vi "Get Compiled Counter And Protection Frames.vi"(0 "XNET Cluster":refnum<k21>, 5 "GUIDs":T9, 7 "Frames per type":T10[](array[typedef]) {"Frame Settings"."Tx Control.Override Period Value Ref" format="%.0x"; "Frame Settings"."Tx Control.Override Period Ref" format="%.0x"; "Frame Settings"."Tx Control.Disable Tx Ref" format="%.0x"; "Frame Settings"."Transmit Trigger Ref" format="%.0x"; "Frame Settings"."Disable Transmission Ref" format="%.0x"; "Frame Refs" format="%.0x"}, 11 "error in (no error)":errorcluster) -> (4 "Frames":T2[](array[typedef]) {"Protection Configurations"."CRC Channels"."Data Type" items=["Signed", "Unsigned", "IEEE Float"]}, 6 "Signals Refs":T1[](array[typedef]) format="%.0x", 8 "Counters and Protection Refs":T1[](array[typedef]) format="%.0x", 10 "Override Refs":T1[](array[typedef]) format="%.0x", 15 "error out":errorcluster)   [LabVIEW 2023, in "Protection and Counter Support System Explorer.lvlib"]
uses:
  Protection and Counter Support System Explorer.lvlib
  Types/Export Frames List and Type.ctl
  Shared/Types/Exported Frame Type.ctl
  <vilib>/NI VeriStand/Custom Device API/Custom Device Item Ref.ctl
  Types/Exported Frame Settings.ctl
  Shared/Types/Exported Event Trigger Type.ctl
  Types/Export Frame GUIDs List.ctl
  Shared/Types/Exported Frame Settings.ctl
  Shared/Types/Exported Protection Settings.ctl
  Shared/Types/Protection Type.ctl
  Shared/Types/XNET Signal Configuration.ctl
  Shared/Types/Exported Counter Settings.ctl
  <vilib>/NI VeriStand/Custom Device Tools/Custom Device Utility Library/NI VeriStand - Search for All Items by GUID.vi
  Shared/Protection and Counter Support Shared.lvlib
  <vilib>/NI VeriStand/Custom Device API/Custom Device API.lvlib
  <resource>/objmgr/xnet.rc
  <vilib>/NI VeriStand/Custom Device Tools/Custom Device Utility Library/Custom Device Utility Library.lvlib
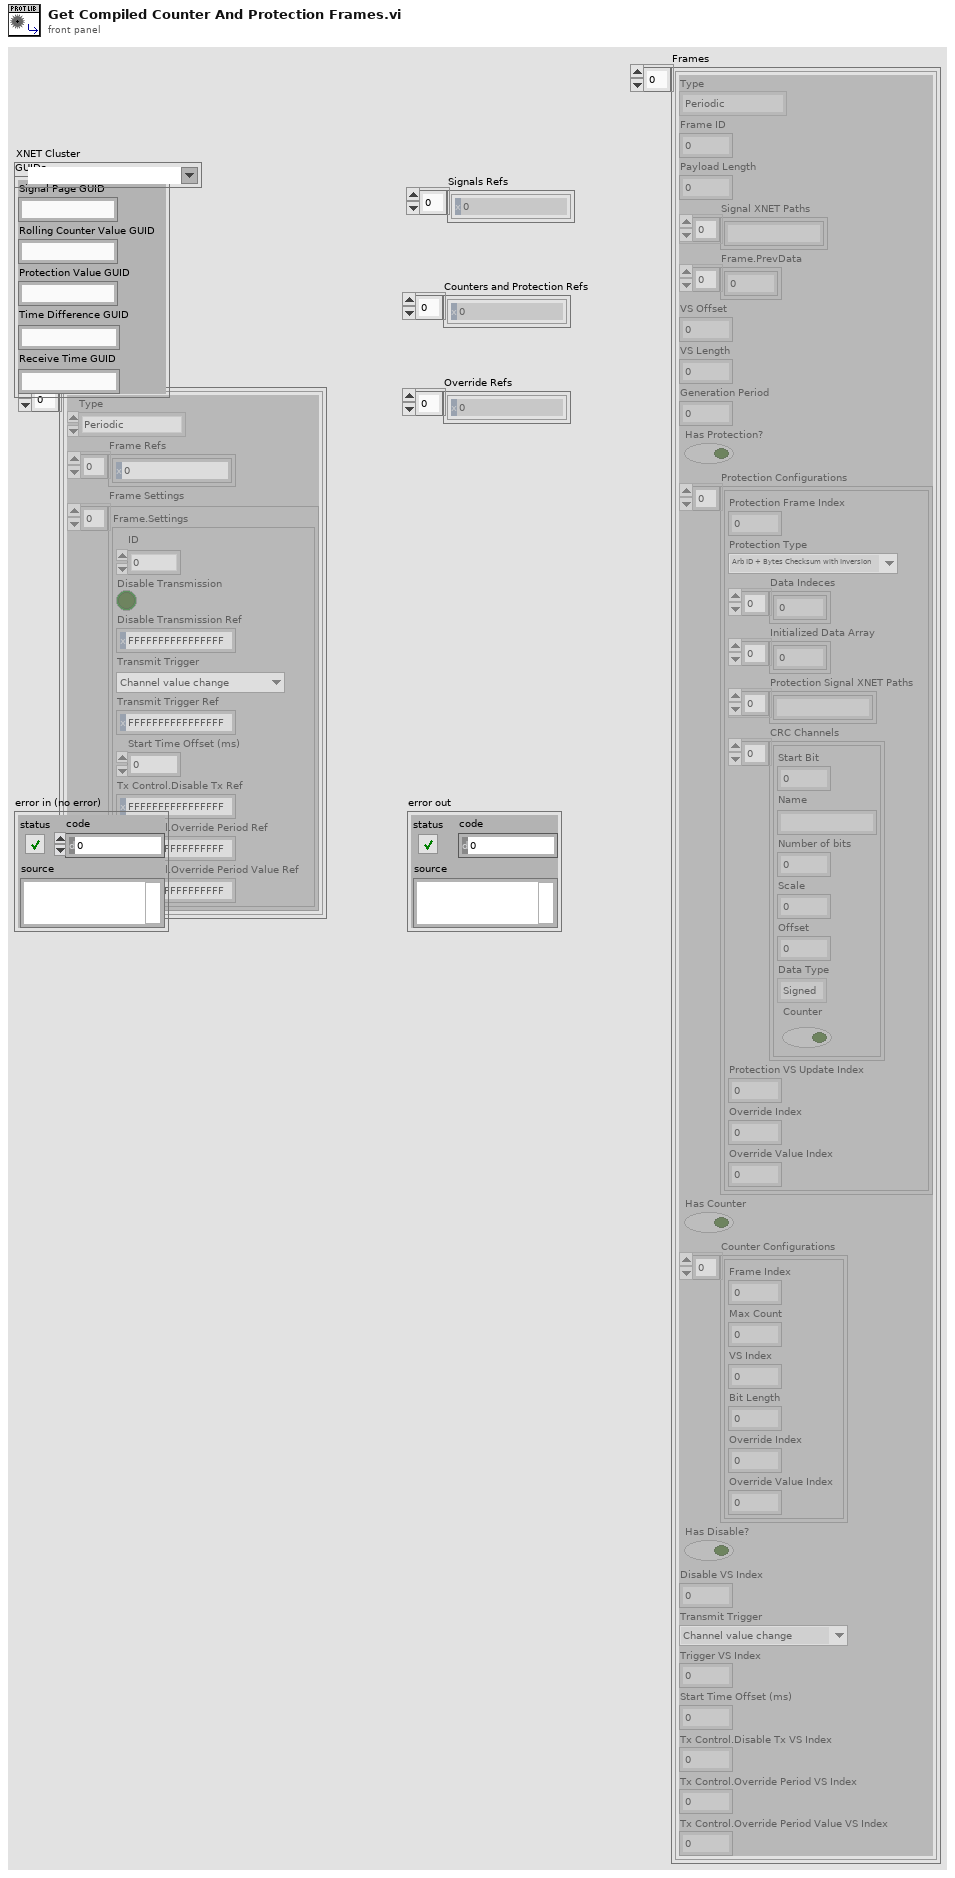
[diagram p1: front panel]
types:
  T1 = typedef "Custom Device API.lvlib/Custom Device Item Ref.ctl" = u64
  T2 = typedef "Protection and Counter Support Shared.lvlib/Exported Frame Settings.ctl" = cluster{"Type":T3, "Frame ID":u32, "Payload Length":u32, "Signal XNET Paths":string[], "Frame.PrevData":dbl[], "VS Offset":i32, "VS Length":i32, "Generation Period":u32, "Has Protection?":bool, "Protection Configurations":T4[], "Has Counter":bool, "Counter Configurations":T7[], "Has Disable?":bool, "Disable VS Index":i32, "Transmit Trigger":T8, "Trigger VS Index":i32, "Start Time Offset (ms)":u32, "Tx Control.Disable Tx VS Index":i32, "Tx Control.Override Period VS Index":i32, "Tx Control.Override Period Value VS Index":i32}
  T3 = typedef "Protection and Counter Support Shared.lvlib/Exported Frame Type.ctl" = enum16{"Periodic", "Event", "Periodic/Event"}
  T4 = typedef "Protection and Counter Support Shared.lvlib/Exported Protection Settings.ctl" = cluster{"Protection Frame Index":i32, "Protection Type":T5, "Data Indeces":i32[], "Initialized Data Array":dbl[], "Protection Signal XNET Paths":string[], "CRC Channels":T6[], "Protection VS Update Index":i32, "Override Index":i32, "Override Value Index":i32}
  T5 = typedef "Protection and Counter Support Shared.lvlib/Protection Type.ctl" = enum16{"Arb ID + Bytes Checksum with Inversion", "Arb ID + Bytes CRC with Inversion", "Reversed Raw Signal Checksum with Inversion", "Concatenated Two's Compliment", "LP_CRC8", "LP_Checksum", "LP_CRC8_MRS"}
  T6 = typedef "Protection and Counter Support Shared.lvlib/XNET Signal Configuration.ctl" = cluster{"Start Bit":i32, "Name":string, "Number of bits":i32, "Scale":dbl, "Offset":dbl, "Data Type":u32, "Counter":bool}
  T7 = typedef "Protection and Counter Support Shared.lvlib/Exported Counter Settings.ctl" = cluster{"Frame Index":i32, "Max Count":dbl, "VS Index":i32, "Bit Length":i64, "Override Index":i32, "Override Value Index":i32}
  T8 = typedef "Protection and Counter Support Shared.lvlib/Exported Event Trigger Type.ctl" = enum16{"Channel value change", "Trigger channel (not zero)", "Channel value change or trigger channel (not zero)", "Trigger channel (any value change)", "Channel value change or trigger channel (any value change)"}
  T9 = typedef "Protection and Counter Support System Explorer.lvlib/Export Frame GUIDs List.ctl" = cluster{"Signal Page GUID":string, "Rolling Counter Value GUID":string, "Protection Value GUID":string, "Time Difference GUID":string, "Receive Time GUID":string}
  T10 = typedef "Protection and Counter Support System Explorer.lvlib/Export Frames List and Type.ctl" = cluster{"Type":T3, "Frame Refs":T1[], "Frame Settings":T11[]}
  T11 = typedef "Protection and Counter Support System Explorer.lvlib/Exported Frame Settings.ctl" = cluster{"ID":u32, "Disable Transmission":bool, "Disable Transmission Ref":T1, "Transmit Trigger":T8, "Transmit Trigger Ref":T1, "Start Time Offset (ms)":u32, "Tx Control.Disable Tx Ref":T1, "Tx Control.Override Period Ref":T1, "Tx Control.Override Period Value Ref":T1}
  T12 = typedef "Custom Device API.lvlib/Custom Device Item Info.ctl" = cluster{"Name":string, "Is Channel":bool, "GUID":string, "Is Waveform":bool}
  T13 = typedef "Protection and Counter Support System Explorer.lvlib/Protection Signal Settings.ctl" = cluster{"Input Channels":T14[], "Protection Type":T5}
  T14 = typedef "Protection and Counter Support System Explorer.lvlib/Protection Signal Linked Channel.ctl" = cluster{"Node Ref":T1}
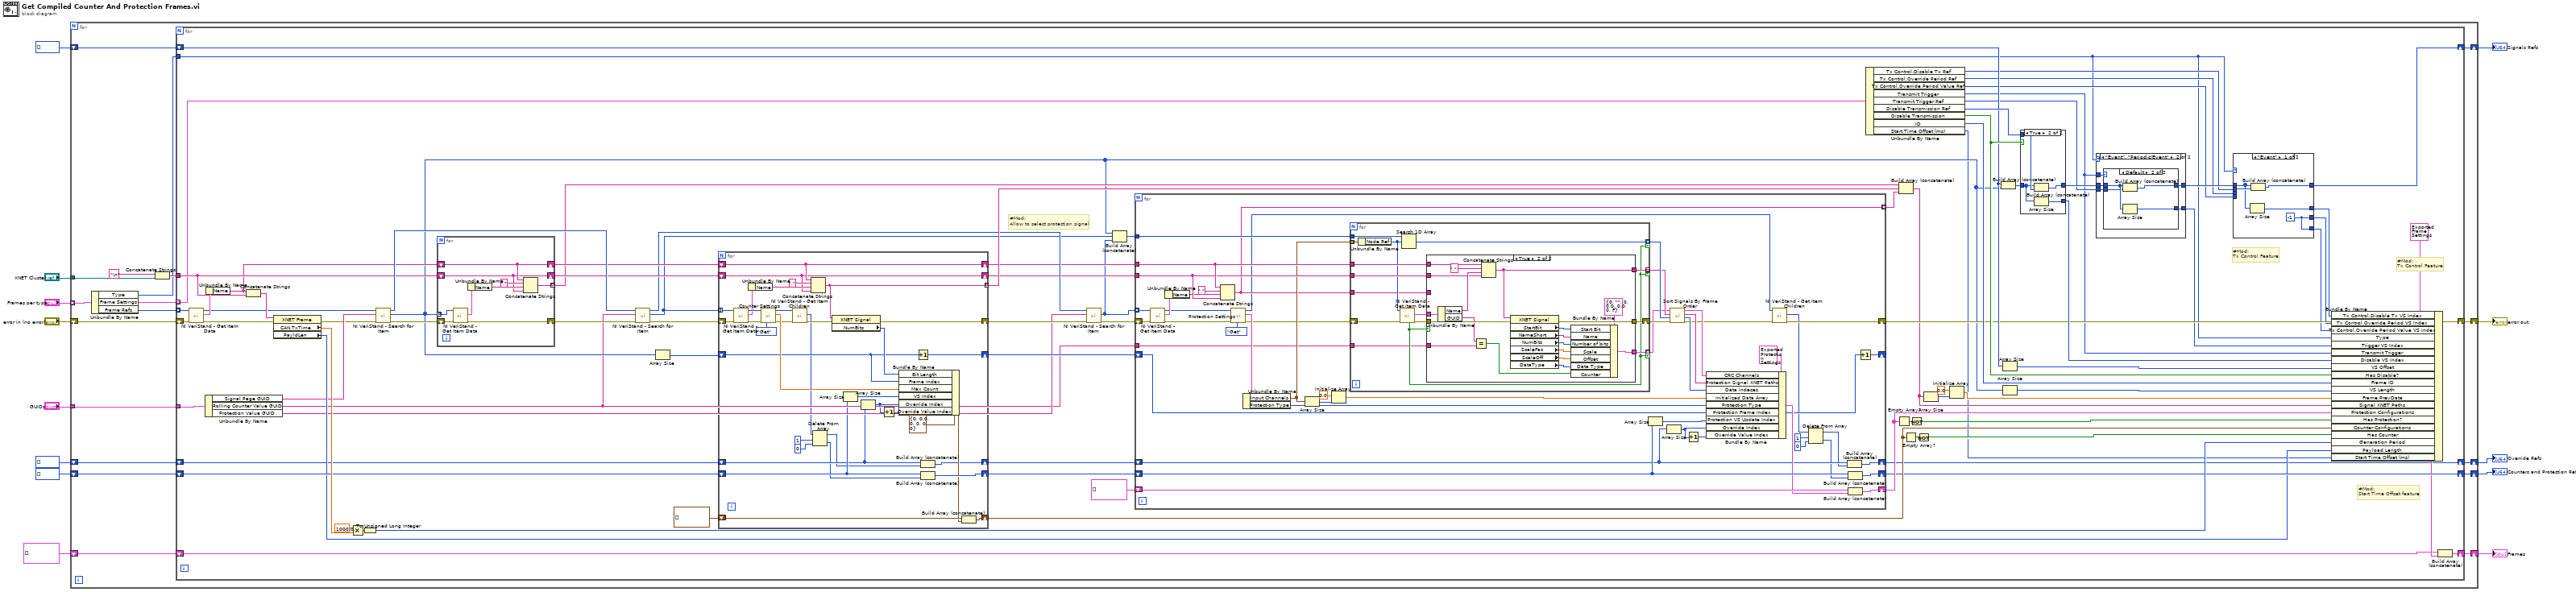
[diagram p0: block diagram]
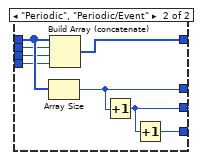
[diagram p2: hidden frame]
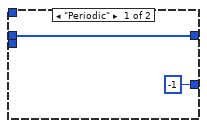
[diagram p3: hidden frame]
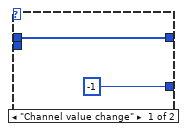
[diagram p4: hidden frame]
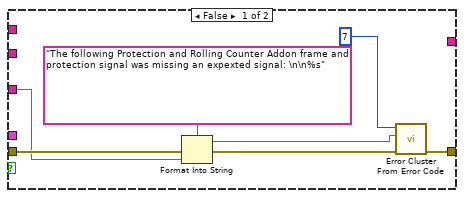
[diagram p5: hidden frame]
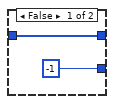
[diagram p6: hidden frame]
diagram:
  n1 = for {
    tunnel: "XNET Cluster" -> [w31]
    shift-right: [w26] -> w1
    shift-left: "error in (no error)" -> [w20]
    shift-right: [w25] -> w7
    shift-left: T2[] [] -> [w24]
    shift-right: [w28] -> w5
    shift-left: T1[] [] -> [w23]
    shift-right: [w27] -> w6
    shift-left: T1[] [] -> [w22]
    tunnel: "GUIDs" -> [w21]
    tunnel: "Frames per type" -> [w19] mode=indexing
    shift-right: [w14] -> w2
    shift-left: T1[] [] -> [w15]
    n2 = Unbundle By Name(w19) -> ("Type"=w18:T3, "Frame Settings"=w16:T11[], "Frame Refs"=w17:T1[])
    n3 = Concatenate Strings("\n", w31) -> (w29:string)
    n4 = for {
      tunnel: w17 -> [w99] mode=indexing
      shift-right: [w69] -> w26
      shift-left: w20 -> [w100]
      shift-right: [w37] -> w28
      shift-left: w23 -> [w109]
      tunnel: w29 -> [w84]
      shift-right: [w63] -> w27
      shift-left: w22 -> [w90]
      shift-right: [w54] -> w25
      shift-left: w24 -> [w53]
      tunnel: w18 -> [w36]
      tunnel: w21 -> [w52]
      tunnel: w16 -> [w49] mode=indexing
      shift-right: [w44] -> w14
      shift-left: w15 -> [w46]
      # "#Mod:\nTx Control Feature"
      # "#Mod:\nTx Control Feature"
      # "#Mod:\nAllow to select protection signal"
      # "#Mod:\nStart Time Offset feature"
      n5 = call <vilib>:"NI VeriStand - Get Item Data.vi"("error in (no error)"=w100, "Item Ref in"=w99) -> ("error out"=w96:errorcluster, "Item Info"=w98:T12, "Item Ref out"=w32:T1)  [unwired: 6 in, 1 out]
      n6 = Unbundle By Name(w52) -> ("Signal Page GUID"=w51:string, "Rolling Counter Value GUID"=w47:string, "Protection Value GUID"=w50:string)
      n7 = Unbundle By Name(w98) -> ("Name"=w83:string)
      n8 = Concatenate Strings(w83, w84) -> (w97:string)
      n9 = property class="XNET Frame"(reference=w97, error in=w96) -> (error out=w48:errorcluster, "CAN.TxTime"=w94:dbl, "PayldLen"=w59:u32)  [unwired: 1 out]
      n10 = Multiply(x=1000.0 ("y"), y=w94) -> (x*y=w95:dbl)
      n11 = To Unsigned Long Integer(number=w95) -> (unsigned 32bit integer=w92:u32)
      n12 = call-poly <vilib>:"NI VeriStand - Search for Item.vi"("error in"=w48, "Item GUID"=w51, "Section Ref in"=w32) -> ("error out"=w86:errorcluster, "Item Refs"=w61:T1[], "Section Ref out"=w89:T1)  [unwired: 5 in, 1 out]
      n13 = for {
        tunnel: w61 -> [w239] mode=indexing
        shift-right: [w233] -> w85
        shift-left: w86 -> [w238]
        tunnel: [w235] -> w80 mode=indexing
        shift-right: [w232] -> w82
        shift-left: w83 -> [w232]
        shift-right: [w231] -> w81
        shift-left: w84 -> [w231]
        n14 = call <vilib>:"NI VeriStand - Get Item Data.vi"("error in (no error)"=w238, "Item Ref in"=w239) -> ("error out"=w233:errorcluster, "Item Info"=w234:T12)  [unwired: 6 in, 2 out]
        n15 = Unbundle By Name(w234) -> ("Name"=w236:string)
        n16 = Concatenate Strings(w232, "." ("string"), w236, w231) -> (w235:string)
      }
      n17 = call-poly <vilib>:"NI VeriStand - Search for Item.vi"("error in"=w85, "Item GUID"=w47, "Section Ref in"=w89) -> ("error out"=w88:errorcluster, "Item Refs"=w60:T1[], "Section Ref out"=w77:T1)  [unwired: 5 in, 1 out]
      n18 = Array Size(array=w61) -> (size(s)=w87:i32)
      n19 = for {
        tunnel: w60 -> [w274] mode=indexing
        shift-right: [w255] -> w78
        shift-left: w88 -> [w273]
        shift-right: [w270] -> w101
        shift-left: T7[] [] -> [w269]
        tunnel: [w254] -> w79 mode=indexing
        shift-right: [w264] -> w64
        shift-left: w90 -> [w265]
        shift-right: [w259] -> w74
        shift-left: w87 -> [w252]
        shift-right: [w258] -> w72
        shift-left: w82 -> [w258]
        shift-right: [w257] -> w73
        shift-left: w81 -> [w257]
        shift-right: [w246] -> w45
        shift-left: w46 -> [w251]
        n20 = call <vilib>:"NI VeriStand - Get Item Data.vi"("error in (no error)"=w273, "Item Ref in"=w274) -> ("error out"=w271:errorcluster, "Item Info"=w266:T12, "Item Ref out"=w272:T1)  [unwired: 6 in, 1 out]
        n21 = Unbundle By Name(w266) -> ("Name"=w267:string)
        n22 = call "Counter Settings.vi"("Action"=enum8{"Get", "Set"}."Get", "error in"=w271, "Parent Ref"=w272) -> ("error out"=w248:errorcluster, "Max Count"=w263:dbl, "Parent Ref Out"=w243:T1)  [unwired: 6 in]
        n23 = call <vilib>:"NI VeriStand - Get Item Children.vi"("error in (no error)"=w248, "Item Ref in"=w243) -> ("error out"=w247:errorcluster, "Child Refs"=w241:T1[])  [unwired: 6 in, 2 out]
        n24 = Concatenate Strings(w258, "." ("string"), w267, w257) -> (w254:string)
        n25 = Delete From Array(array=w241, length=1, index=0) -> (deleted portion=w242:T1[], array with subset deleted=w240:T1[])
        n26 = property class="XNET Signal"(reference=w254, error in=w247) -> (error out=w255:errorcluster, "NumBits"=w253:u32)  [unwired: 1 out]
        n27 = Array Size(array=w265) -> (size(s)=w260:i32)
        n28 = Array Size(array=w251) -> (size(s)=w250:i32)
        n29 = Increment(x=w250) -> (x+1=w249:i32)
        n30 = Bundle By Name(cluster=T7 {"Frame Index"=0, "Max Count"=0.0, "VS Index"=0, "Bit Length"=0, "Override Index"=0, "Override Value Index"=0} ("Cluster"), "Bit Length"=w253, "Frame Index"=w252, "Max Count"=w263, "VS Index"=w260, "Override Index"=w250, "Override Value Index"=w249) -> (w262:T7)
        n31 = Increment(x=w252) -> (x+1=w259:i32)
        n32 = Build Array (concatenate)(w251, w240) -> (w246:T1[])
        n33 = Build Array (concatenate)(w265, w242) -> (w264:T1[])
        n34 = Build Array (concatenate)(w269, w262) -> (w270:T7[])
      }
      n35 = call-poly <vilib>:"NI VeriStand - Search for Item.vi"("error in"=w78, "Item GUID"=w50, "Section Ref in"=w77) -> ("error out"=w76:errorcluster, "Item Refs"=w42:T1[])  [unwired: 5 in, 2 out]
      n36 = Build Array (concatenate)(w61, w60, w42) -> (w62:T1[])
      n37 = for {
        tunnel: w42 -> [w189] mode=indexing
        shift-right: [w148] -> w69
        shift-left: w76 -> [w188]
        shift-right: [w185] -> w70
        shift-left: T4[] [] -> [w187]
        tunnel: w62 -> [w186]
        tunnel: w72 -> [w183]
        tunnel: [w165] -> w71 mode=indexing
        shift-right: [w179] -> w63
        shift-left: w64 -> [w180]
        shift-right: [w167] -> _
        shift-left: w74 -> [w168]
        tunnel: w73 -> [w182]
        tunnel: w47 -> [w163]
        shift-right: [w153] -> w44
        shift-left: w45 -> [w152]
        n38 = call <vilib>:"NI VeriStand - Get Item Data.vi"("error in (no error)"=w188, "Item Ref in"=w189) -> ("error out"=w151:errorcluster, "Item Info"=w181:T12, "Item Ref out"=w150:T1)  [unwired: 6 in, 1 out]
        n39 = Unbundle By Name(w181) -> ("Name"=w166:string)
        n40 = Concatenate Strings(w183, "." ("string"), w166, w182) -> (w165:string)
        n41 = call "Protection Settings.vi"("Action"=enum8{"Get", "Set"}."Get", "error in"=w151, "Parent Ref"=w150) -> ("error out"=w171:errorcluster, "Selected Channels"=w178:T13, "Parent Ref Out"=w147:T1)  [unwired: 6 in]
        n42 = Unbundle By Name(w178) -> ("Input Channels"=w176:T14[], "Protection Type"=w177:T5)
        n43 = Array Size(array=w176) -> (size(s)=w175:i32)
        n44 = Initialize Array(0.0 ("element"), w175) -> (w173:dbl[])
        n45 = for {
          tunnel: w186 -> [w194]
          tunnel: w176 -> [w204] mode=indexing
          tunnel: [w203] -> w162 mode=indexing if=w192
          shift-right: [w197] -> w160
          shift-left: w171 -> [w202]
          tunnel: w183 -> [w200]
          tunnel: w182 -> [w199]
          tunnel: [w195] -> w159 mode=indexing if=w192
          tunnel: [w196] -> w158 mode=indexing if=w192
          tunnel: w165 -> [w191]
          tunnel: w163 -> [w190]
          n46 = Unbundle By Name(w204) -> ("Node Ref"=w193:T1)
          n47 = call <vilib>:"NI VeriStand - Get Item Data.vi"("error in (no error)"=w202, "Item Ref in"=w193) -> ("error out"=w198:errorcluster, "Item Info"=w201:T12, "Found"=w192:bool)  [unwired: 6 in, 1 out]
          n48 = Search 1D Array(1D array=w194, element=w193) -> (index of element=w203:i32)  [unwired: 1 in]
          n49 = case shown="True" w192 {
            tunnel: w201 -> [_ w230]
            tunnel: w200 -> [_ w227]
            tunnel: w199 -> [_ w226]
            tunnel: w198 -> [w209 w225]
            tunnel: [w211 w224] -> w197
            tunnel: [_ w216] -> w196
            tunnel: [_ w212] -> w195
            tunnel: w191 -> [w206 _]
            tunnel: w190 -> [_ w215]
            frame False {
              n50 = Format Into String(format string="The following Protection and Rolling Counter Addon frame and protection signal was missing an expexted signal: \n\n%s" ("error message (\"\")"), error in=w209, w206) -> (resulting string=w205:string, error out=w208:errorcluster)  [unwired: 1 in]
              n51 = call <vilib>:"Error Cluster From Error Code.vi"("error in (no error)"=w208, "error message (\"\")"=w205, "error code (0)"=7) -> ("error out"=w211:errorcluster)  [unwired: 6 in]
            }
            frame True {
              n52 = Unbundle By Name(w230) -> ("Name"=w228:string, "GUID"=w213:string)
              n53 = Equal?(x=w213, y=w215) -> (x = y?=w214:bool)
              n54 = Concatenate Strings(w227, "." ("string"), w228, w226) -> (w212:string)
              n55 = property class="XNET Signal"(reference=w212, error in=w225) -> (error out=w224:errorcluster, "StartBit"=w217:u32, "NameShort"=w218:string, "NumBits"=w219:u32, "ScaleFac"=w220:dbl, "ScaleOff"=w221:dbl, "DataType"=w222:u32)  [unwired: 1 out]
              n56 = Bundle By Name(cluster=T6 {"Start Bit"=0, "Name"="", "Number of bits"=0, "Scale"=0.0, "Offset"=0.0, "Data Type"=0, "Counter"=FALSE} ("MonitoredChannelSettings"), "Start Bit"=w217, "Name"=w218, "Number of bits"=w219, "Scale"=w220, "Offset"=w221, "Data Type"=w222, "Counter"=w214) -> (w216:T6)
            }
          }
        }
        n57 = Array Size(array=w180) -> (size(s)=w169:i32)
        n58 = Array Size(array=w152) -> (size(s)=w155:i32)
        n59 = call "Sort Signals By Frame Order.vi"("error in (no error)"=w160, "Node Refs"=w162, "XNET Paths"=w159, "Signals"=w158) -> ("error out"=w149:errorcluster, "Ordered Node Refs"=w161:i32[], "Ordered XNET Paths"=w156:string[], "Ordered Signals"=w157:T6[])  [unwired: 4 in]
        n60 = Increment(x=w155) -> (x+1=w154:i32)
        n61 = Bundle By Name(cluster=T4 {"Protection Frame Index"=0, "Protection Type"=enum."Arb ID + Bytes Checksum with Inversion", "Data Indeces"=[], "Initialized Data Array"=[], "Protection Signal XNET Paths"=[], "CRC Channels"=[], "Protection VS Update Index"=0, "Override Index"=0, "Override Value Index"=0} ("Cluster"), "CRC Channels"=w157, "Protection Signal XNET Paths"=w156, "Data Indeces"=w161, "Initialized Data Array"=w173, "Protection Type"=w177, "Protection Frame Index"=w168, "Protection VS Update Index"=w169, "Override Index"=w155, "Override Value Index"=w154) -> (w172:T4)
        n62 = call <vilib>:"NI VeriStand - Get Item Children.vi"("error in (no error)"=w149, "Item Ref in"=w147) -> ("error out"=w148:errorcluster, "Child Refs"=w143:T1[])  [unwired: 6 in, 2 out]
        n63 = Delete From Array(array=w143, length=1, index=0) -> (deleted portion=w144:T1[], array with subset deleted=w142:T1[])
        n64 = Build Array (concatenate)(w152, w142) -> (w153:T1[])
        n65 = Build Array (concatenate)(w180, w144) -> (w179:T1[])
        n66 = Build Array (concatenate)(w187, w172) -> (w185:T4[])
        n67 = Increment(x=w168) -> (x+1=w167:i32)
      }
      n68 = Unbundle By Name(w49) -> ("Tx Control.Disable Tx Ref"=w40:T1, "Tx Control.Override Period Ref"=w39:T1, "Tx Control.Override Period Value Ref"=w38:T1, "Transmit Trigger"=w57:T8, "Transmit Trigger Ref"=w58:T1, "Disable Transmission Ref"=w112:T1, "Disable Transmission"=w113:bool, "ID"=w114:u32, "Start Time Offset (ms)"=w43:u32)
      n69 = Empty Array?(array=w70) -> (empty?=w103:bool)
      n70 = Build Array (concatenate)(w80, w79, w71) -> (w68:string[])
      n71 = Empty Array?(array=w101) -> (empty?=w105:bool)
      n72 = Not(x=w103) -> (.not. x?=w102:bool)
      n73 = Not(x=w105) -> (.not. x?=w104:bool)
      n74 = Array Size(array=w68) -> (size(s)=w66:i32)
      n75 = Initialize Array(0.0 ("element"), w66) -> (w65:dbl[])
      n76 = Build Array (concatenate)(w109, w61) -> (w110:T1[])
      n77 = Array Size(array=w109) -> (size(s)=w108:i32)
      n78 = Array Size(array=w61) -> (size(s)=w91:i32)
      n79 = case shown="True" w113 {
        tunnel: w110 -> [w276 w278]
        tunnel: [w276 w280] -> w111
        tunnel: w112 -> [_ w279]
        tunnel: [-1 w277] -> w107
        frame False {
        }
        frame True {
          n80 = Build Array (concatenate)(w278, w279) -> (w280:T1[])
          n81 = Array Size(array=w278) -> (size(s)=w277:i32)
        }
      }
      n82 = case shown="\"Event\", \"Periodic/Event\"" w36 {
        tunnel: w111 -> [w130 w135]
        tunnel: [w130 w134] -> w41
        tunnel: w58 -> [_ w133]
        tunnel: w57 -> [_ w132]
        tunnel: [-1 w131] -> w56
        frame "Periodic" {
        }
        frame "Event", "Periodic/Event" {
          n83 = case shown="Default" w132 {
            tunnel: w135 -> [w137 w140]
            tunnel: [w137 w141] -> w134
            tunnel: [-1 w139] -> w131
            tunnel: w133 -> [_ w138]
            frame "Channel value change" {
            }
            frame Default {
              n84 = Array Size(array=w140) -> (size(s)=w139:i32)
              n85 = Build Array (concatenate)(w140, w138) -> (w141:T1[])
            }
          }
        }
      }
      n86 = case shown="\"Event\"" w36 {
        tunnel: w41 -> [w118 w128]
        tunnel: [w120 w127] -> w37
        tunnel: w40 -> [w119 w126]
        tunnel: [w117 w123] -> w35
        tunnel: w39 -> [_ w125]
        tunnel: w38 -> [_ w124]
        tunnel: [w116 w122] -> w34
        tunnel: [w116 w121] -> w33
        frame "Event" {
          w116 = -1
          n87 = Array Size(array=w118) -> (size(s)=w117:i32)
          n88 = Build Array (concatenate)(w118, w119) -> (w120:T1[])
        }
        frame "Periodic", "Periodic/Event" {
          n89 = Array Size(array=w128) -> (size(s)=w123:i32)
          n90 = Build Array (concatenate)(w128, w126, w125, w124) -> (w127:T1[])
          n91 = Increment(x=w123) -> (x+1=w122:i32)
          n92 = Increment(x=w122) -> (x+1=w121:i32)
        }
      }
      n93 = Bundle By Name(cluster=T2 {"Type"=enum."Periodic", "Frame ID"=0, "Payload Length"=0, "Signal XNET Paths"=[], "Frame.PrevData"=[], "VS Offset"=0, "VS Length"=0, "Generation Period"=0, "Has Protection?"=FALSE, "Protection Configurations"=[], "Has Counter"=FALSE, "Counter Configurations"=[], "Has Disable?"=FALSE, "Disable VS Index"=0, "Transmit Trigger"=enum."Channel value change", "Trigger VS Index"=0, "Start Time Offset (ms)"=0, "Tx Control.Disable Tx VS Index"=0, "Tx Control.Override Period VS Index"=0, "Tx Control.Override Period Value VS Index"=0} ("Frame Settings"), "Tx Control.Disable Tx VS Index"=w35, "Tx Control.Override Period VS Index"=w34, "Tx Control.Override Period Value VS Index"=w33, "Type"=w36, "Trigger VS Index"=w56, "Transmit Trigger"=w57, "Disable VS Index"=w107, "VS Offset"=w108, "Has Disable?"=w113, "Frame ID"=w114, "VS Length"=w91, "Frame.PrevData"=w65, "Signal XNET Paths"=w68, "Protection Configurations"=w70, "Has Protection?"=w102, "Counter Configurations"=w101, "Has Counter"=w104, "Generation Period"=w92, "Payload Length"=w59, "Start Time Offset (ms)"=w43) -> (w55:T2)
      n94 = Build Array (concatenate)(w53, w55) -> (w54:T2[])
    }
  }
  "Frames" <- w7
  "error out" <- w1
  "Counters and Protection Refs" <- w6
  "Signals Refs" <- w5
  "Override Refs" <- w2
